vi "GetAvailableBackends.vi"(8 "error in":errorcluster) -> (0 "error out":errorcluster, 3 "Backends":T1[](array[typedef]))   [LabVIEW 2020, in "OpenLvVision_OpenCv.lvlib"]
doc: "Retruns the available backends and its targets"
uses:
  OpenLvVision_OpenCv.lvlib
  TypeDef/BackenTarget.ctl
  TypeDef/Backend.ctl
  TypeDef/Target.ctl
  Dlls/OlvOpenCvWrapper.dll
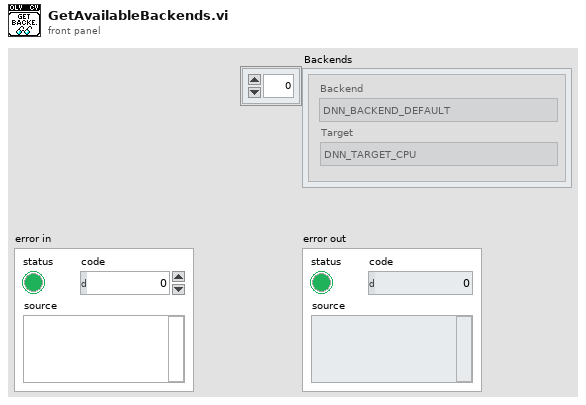
[diagram p1: front panel]
types:
  T1 = typedef "OpenLvVision_OpenCv.lvlib/BackenTarget.ctl" = cluster{"Backend":T2, "Target":T3}
  T2 = typedef "OpenLvVision_OpenCv.lvlib/Backend.ctl" = enum16{"DNN_BACKEND_DEFAULT", "DNN_BACKEND_HALIDE", "DNN_BACKEND_INFERENCE_ENGINE", "DNN_BACKEND_OPENCV", "DNN_BACKEND_VKCOM", "DNN_BACKEND_CUDA", "DNN_BACKEND_WEBNN", "DNN_BACKEND_TIMVX", "DNN_BACKEND_CANN"}
  T3 = typedef "OpenLvVision_OpenCv.lvlib/Target.ctl" = enum16{"DNN_TARGET_CPU", "DNN_TARGET_OPENCL", "DNN_TARGET_OPENCL_FP16", "DNN_TARGET_MYRIAD", "DNN_TARGET_VULKAN", "DNN_TARGET_FPGA", "DNN_TARGET_CUDA", "DNN_TARGET_CUDA_FP16", "DNN_TARGET_HDDL", "DNN_TARGET_NPU", "DNN_TARGET_CPU_FP16"}
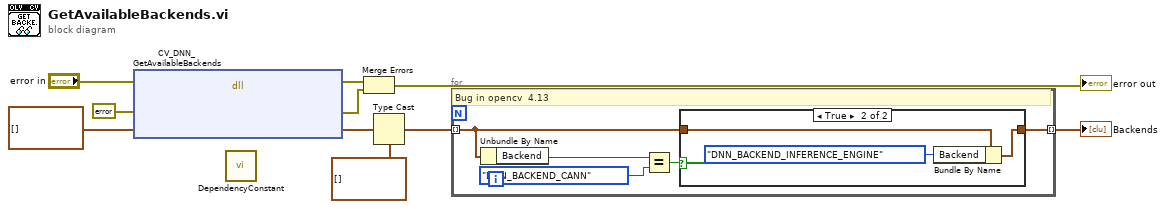
[diagram p0: block diagram]
diagram:
  n1 = dll-call lib="C:/Users/lukas/Downloads/OpenLvVision_OpenCv/SourceCode/LabView/OpenLvVision_OpenCv/Dlls/OlvOpenCvWrapper.dll" fn="CV_DNN_GetAvailableBackends"(error in="error in", "Error"=errorcluster {"status"=FALSE, "code"=0, "source"=""} ("error out"), "backendArrayHandle"=T1[] []) -> (error out=w9:errorcluster, "Error"=w7:errorcluster, "backendArrayHandle"=w3:T1[])  [unwired: 3 in, 1 out]
  n2 = call "DependencyConstant.vi"() -> ()  [unwired: 12 in]
  n3 = Merge Errors(w9, w7) -> (→"error out":errorcluster)
  n4 = Type Cast(type=T1[] [], x=w3) -> (*(type *) &x=w2:T1[])
  n5 = for {
    tunnel: w2 -> [w12] mode=indexing
    tunnel: [w11] -> w4 mode=indexing
    # "Bug in opencv  4.13"
    n6 = Unbundle By Name(w12) -> ("Backend"=w15:T2)
    n7 = Equal?(x=w15, y=Backend."DNN_BACKEND_CANN" ("Backend")) -> (x = y?=w13:bool)
    n8 = case shown="True" w13 {
      tunnel: w12 -> [w16 w19]
      tunnel: [w16 w18] -> w11
      frame False {
      }
      frame True {
        n9 = Bundle By Name(cluster=w19, "Backend"=Backend."DNN_BACKEND_INFERENCE_ENGINE") -> (w18:T1)
      }
    }
  }
  "Backends" <- w4
